vi "MB Read Coil.vi"(8 "error in (no error)":errorcluster, 9 "Key":string, 11 "Devices":T1) -> (0 "error out":errorcluster, 2 "coils":bool, 3 "Devices out":T1)   [LabVIEW 2021]
uses:
  Modbus Cluster.ctl
  <vilib>/NI/Modbus Library/API/Master/Modbus Master.lvclass
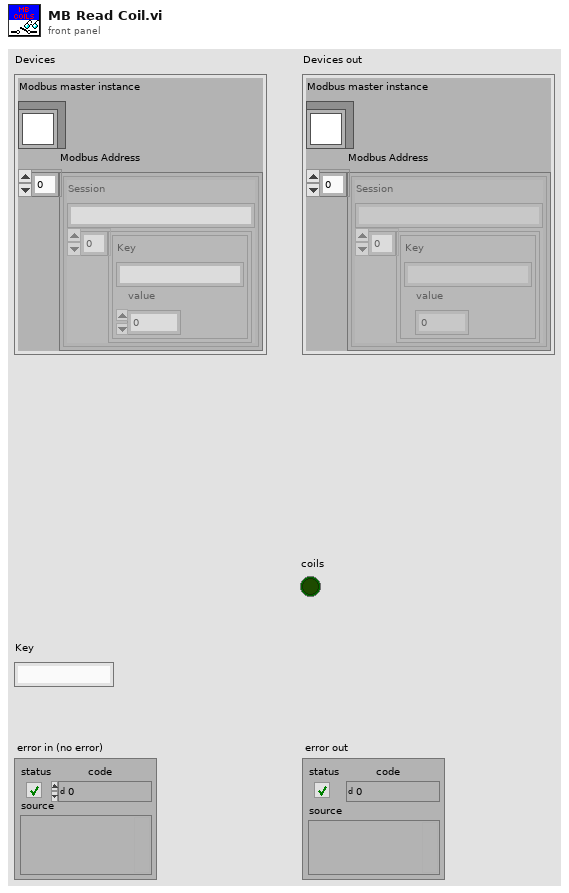
[diagram p1: front panel]
types:
  T1 = typedef "Modbus Cluster.ctl" = cluster{"Modbus master instance":refnum<class "Modbus Master.lvclass">, "Modbus Address":cluster{"Session":string, cluster{"Key":string, "value":u32}[]}[]}
  T2 = cluster{"Session":string, cluster{"Key":string, "value":u32}[]}[]
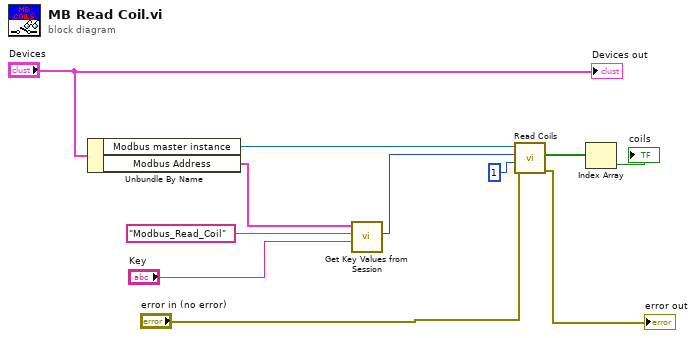
[diagram p0: block diagram]
diagram:
  n1 = Unbundle By Name("Devices") -> ("Modbus master instance"=w11:refnum<class "Modbus Master.lvclass">, "Modbus Address"=w8:T2)
  n2 = call "Get Key Values from Session.vi"("Key"="Key", "Session"="Modbus_Read_Coil", "Ini File"=w8) -> ("Search Key Value"=w3:u32)  [unwired: 6 in, 2 out]
  n3 = call-dynamic "Read Coils.vi"("error in"="error in (no error)", "number of inputs"=u16 1, "starting address"=w3, "Modbus master in"=w11) -> ("error out"=→"error out":errorcluster, "coils"=w2:bool[])  [unwired: 5 in, 1 out]
  n4 = Index Array(array=w2) -> (element=→"coils":bool)  [unwired: 1 in]
  "Devices out" <- "Devices"
